vi "Read_EOS_BOS_ID.vi"(0 "Beam in":refnum<class "Beam.lvclass">, 11 "error in (no error)":errorcluster) -> (3 "Read Status":bool, 4 "Beam out":refnum<class "Beam.lvclass">, 6 "Spill ID":i32, 8 "BOS Time":dbl format="%#.6f", 10 "EOS Time":dbl format="%#.6f", 15 "error out":errorcluster)   [LabVIEW 2019, in "Beam.lvclass"]
uses:
  Beam.lvclass
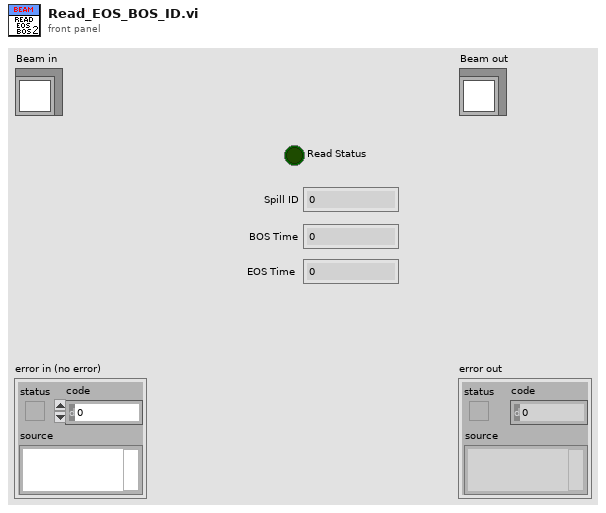
[diagram p1: front panel]
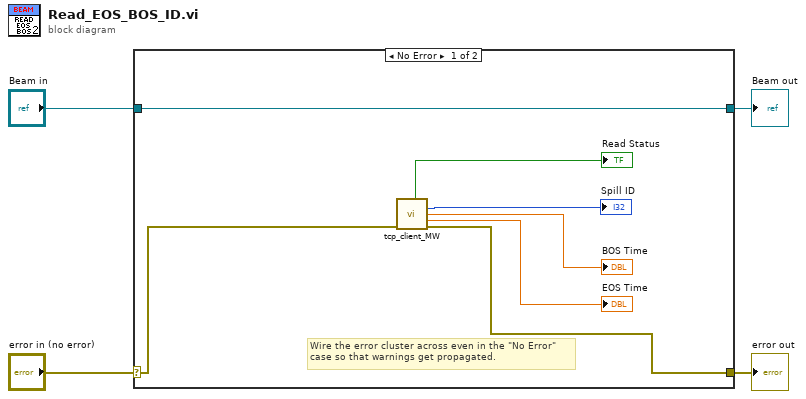
[diagram p0: block diagram]
diagram:
  n1 = case shown="No Error" "error in (no error)" {
    selector: "error in (no error)" -> [w7 w13]
    tunnel: [w6 w13] -> w3
    tunnel: [w11 w12] -> w1
    tunnel: "Beam in" -> [w11 w12]
    frame No Error {
      # "Wire the error cluster across even in the \"No Error\"\ncase so that warnings get propagated."
      n2 = call "tcp_client_MW.vi"("error in"=w7) -> ("status"=→"Read Status":bool, "Spill ID"=→"Spill ID":i32, "BOS Time"=→"BOS Time":dbl, "EOS Time"=→"EOS Time":dbl, "error out"=w6:errorcluster)  [unwired: 9 in, 1 out]
    }
    frame Error {
    }
  }
  "error out" <- w3
  "Beam out" <- w1
